vi "readSetting.vi"(8 "error in (no error)":errorcluster, 10 "Config File Name":string="optiPSSN_x00.ctrl", 11 "OptCtrl in":refnum<class "OptCtrl.lvclass">) -> (0 "error out":errorcluster, 3 "OptCtrl out":refnum<class "OptCtrl.lvclass">)   [LabVIEW 2016, in "OfcFunc.lvlib" / "OptCtrl.lvclass"]
doc: "Read the configuration setting file of optimal control."
uses:
  OptCtrl.lvclass
  OptCtrl.lvclass/OptCtrl.ctl
  MatOper/MatOper.lvclass
panel:
  in  "Parameter List":string[](array[string])=["control_strategy", "xref", "M1M3_actuator_penalty", "M2_actuator_penalty", "Motion_penalty"]
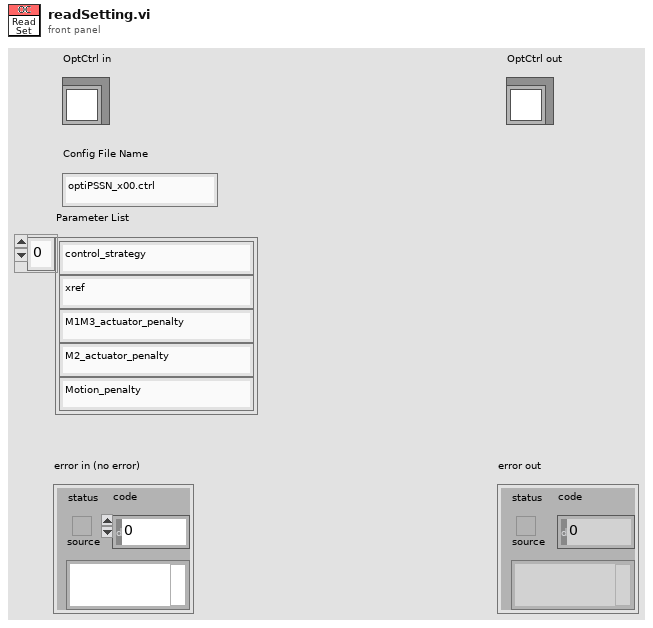
[diagram p1: front panel]
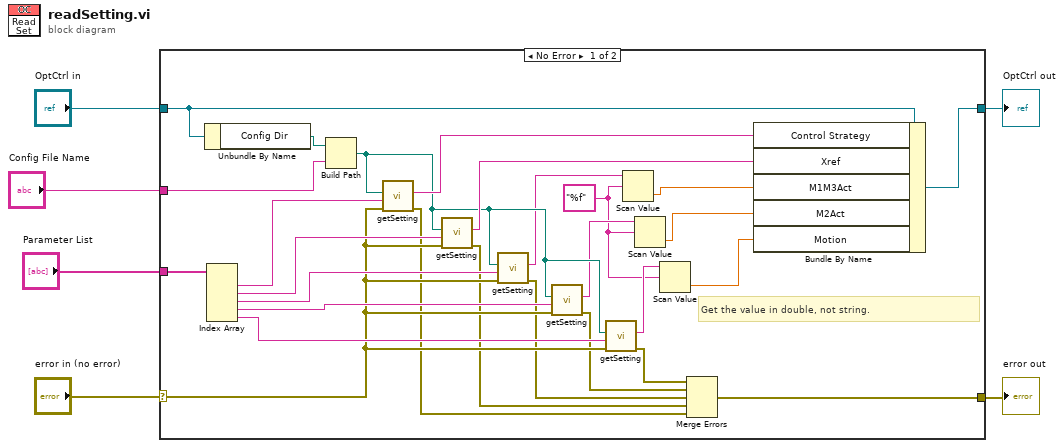
[diagram p0: block diagram]
diagram:
  n1 = case shown="No Error" "error in (no error)" {
    selector: "error in (no error)" -> [w13 w35]
    tunnel: [w7 w35] -> w5
    tunnel: [w28 w34] -> w3
    tunnel: "OptCtrl in" -> [w29 w34]
    tunnel: "Config File Name" -> [w32 _]
    tunnel: "Parameter List" -> [w31 _]
    frame No Error {
      w14 = "%f" ("format string")
      # "Get the value in double, not string."
      n2 = Unbundle By Name(w29) -> ("Config Dir"=w33:path)
      n3 = Index Array(array=w31) -> (element #1=w30:string, element #2=w26:string, element #3=w24:string, element #4=w22:string, element #5=w21:string)  [unwired: 5 in]
      n4 = Build Path(base path=w33, name or relative path=w32) -> (appended path=w23:path)
      n5 = call "getSetting.vi"("error in (no error)"=w13, "Parameter"=w30, "Path"=w23) -> ("error out"=w8:errorcluster, "Value"=w27:string)  [unwired: 6 in, 1 out]
      n6 = call "getSetting.vi"("error in (no error)"=w13, "Parameter"=w26, "Path"=w23) -> ("error out"=w9:errorcluster, "Value"=w25:string)  [unwired: 6 in, 1 out]
      n7 = call "getSetting.vi"("error in (no error)"=w13, "Parameter"=w24, "Path"=w23) -> ("error out"=w10:errorcluster, "Value"=w18:string)  [unwired: 6 in, 1 out]
      n8 = call "getSetting.vi"("error in (no error)"=w13, "Parameter"=w22, "Path"=w23) -> ("error out"=w11:errorcluster, "Value"=w16:string)  [unwired: 6 in, 1 out]
      n9 = call "getSetting.vi"("error in (no error)"=w13, "Parameter"=w21, "Path"=w23) -> ("error out"=w12:errorcluster, "Value"=w20:string)  [unwired: 6 in, 1 out]
      n10 = Scan Value(string=w18, format string=w14) -> (value=w17:dbl)  [unwired: 1 in, 1 out]
      n11 = Scan Value(string=w16, format string=w14) -> (value=w15:dbl)  [unwired: 1 in, 1 out]
      n12 = Scan Value(string=w20, format string=w14) -> (value=w19:dbl)  [unwired: 1 in, 1 out]
      n13 = Merge Errors(w12, w11, w10, w9, w8) -> (w7:errorcluster)
      n14 = Bundle By Name(cluster=w29, "Control Strategy"=w27, "Xref"=w25, "M1M3Act"=w17, "M2Act"=w15, "Motion"=w19) -> (w28:refnum<class "OptCtrl.lvclass">)
    }
    frame Error {
    }
  }
  "error out" <- w5
  "OptCtrl out" <- w3
